vi "Test Cfg Read.vi"() -> ()   [LabVIEW 2012]
uses:
  Reusable/CRDS/Main/CRDS.lvclass
  CRDS Class/Main Class/CRDS.lvclass
panel:
  out "error out 4":errorcluster
  out "error out 3":errorcluster
  out "error out 2":errorcluster
  out "error out":errorcluster
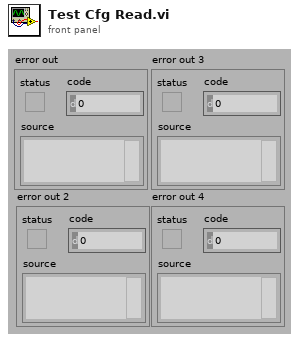
[diagram p1: front panel]
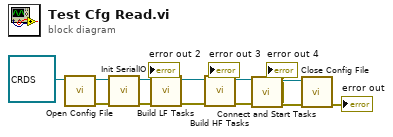
[diagram p0: block diagram]
diagram:
  n1 = call "Open Config File.vi"("CRDS in"=refnum<class "CRDS.lvclass"> refnum) -> ("error out"=w6:errorcluster, "CRDS out"=w12:refnum<class "CRDS.lvclass">)  [unwired: 9 in]
  n2 = call "Init SerialIO.vi"("error in"=w6, "CRDS in"=w12) -> ("error out"=→"error out 2":errorcluster, "CRDS out"=w11:refnum<class "CRDS.lvclass">)  [unwired: 7 in, 1 out]
  n3 = call "Build LF Tasks.vi"("CRDS in"=w11) -> ("error out"=→"error out 3":errorcluster, "CRDS out"=w10:refnum<class "CRDS.lvclass">)  [unwired: 9 in]
  n4 = call "Build HF Tasks.vi"("CRDS in"=w10) -> ("error out"=→"error out 4":errorcluster, "CRDS out"=w9:refnum<class "CRDS.lvclass">)  [unwired: 9 in]
  n5 = call "Connect and Start Tasks.vi"("CRDS in"=w9) -> ("error out"=w5:errorcluster, "CRDS out"=w8:refnum<class "CRDS.lvclass">)  [unwired: 9 in]
  n6 = call "Close Config File.vi"("error in"=w5, "CRDS in"=w8) -> ("error out"=→"error out":errorcluster)  [unwired: 8 in, 1 out]
